vi "niUSRP EX Rx Continuous Async.vi"() -> ()   [LabVIEW 2020]
doc: "Continuously acquires a communication signal that starts immediately. The device is not synchronized to external Reference Clocks or timebases."
uses:
  <instrlib>/niUSRP/niUSRP Timestamp.ctl
  <extravilib>/ChannelInstances/High Speed Stream-a[.](cdb)/_Read For Replicate.vi
  <extravilib>/ChannelInstances/High Speed Stream-a[.](cdb)/Instantiate.vi
  <extravilib>/ChannelInstances/High Speed Stream-a[.](cdb)/)Channel.vi
  <extravilib>/ChannelInstances/High Speed Stream-a[.](cdb)/Abort Signal/Init Signal.vi
  <instrlib>/niUSRP/niUSRP Fetch Rx Data (CDB WDT).vi
  <vilib>/measure/maspectr.llb/FFT Power Spectrum for 1 Chan (CDB).vi
  <vilib>/measure/NI_MAPro.lvlib
  <extravilib>/ChannelInstances/High Speed Stream-a[.](cdb).lvlib
panel:
  out "size(s)":i32
  out "element":cdb[](array[numeric])
  out "error out":errorcluster
  in  "Enabled Channel":string="0"
  out "Actual Rx Timestamp":T1
  in  "Stop":bool
  in  "Device Name":refnum<k15>="192.168.10.2"
  in  "Active Antenna":string="RX1"
  out "Baseband Power Spectrum":cluster{"f0":dbl, "df":dbl, "magnitude":dbl[]}(graph)
  in  "Timeout":dbl=10.0 format="%#.3ps"
  in  "Number of Samples":i64=16384
  out "IQ Graph":waveform(dbl)[](graph)
  out "Coerced Gain":dbl format="%#_6f"
  out "Coerced Carrier Frequency":dbl=100000.0 format="%#_6p"
  out "Coerced IQ Rate [S/sec]":dbl=100000.0 format="%#_6p"
  in  "Gain":dbl=1.0 format="%#_6f"
  in  "Carrier Frequency":dbl=2000000000.0 format="%#_6p"
  in  "IQ Rate [S/sec]":dbl=1000000.0 format="%#_6p"
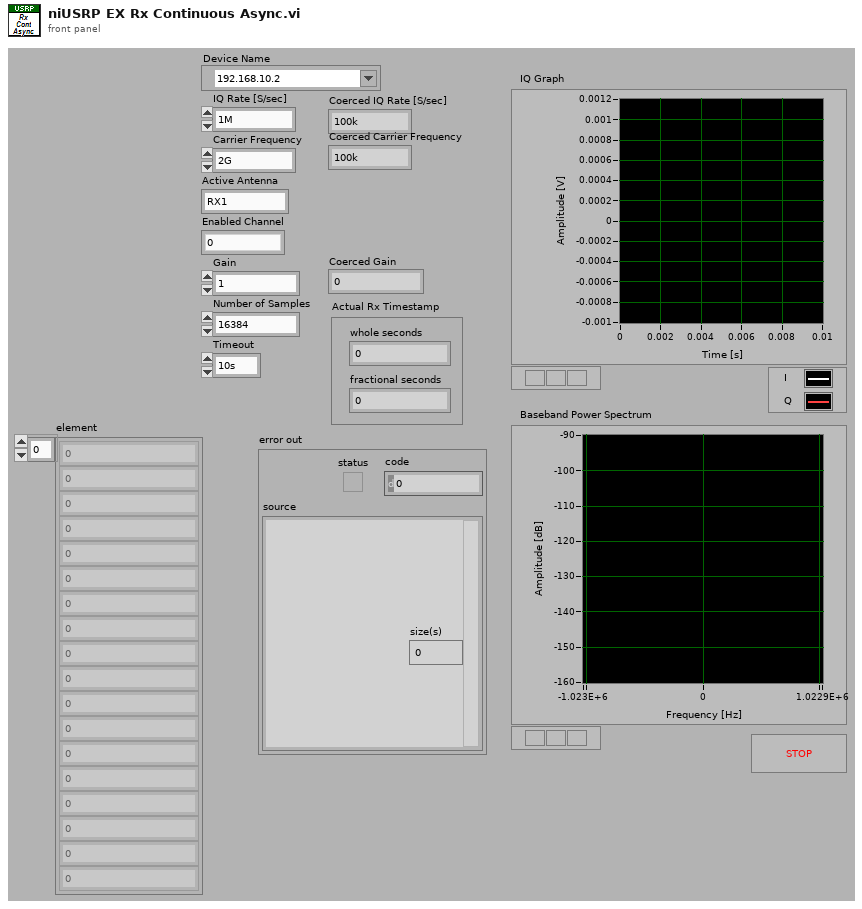
[diagram p1: front panel]
types:
  T1 = typedef "niUSRP Timestamp.ctl" = cluster{"whole seconds":u64, "fractional seconds":dbl}
  T2 = typedef "High Speed Stream-a[.](cdb).lvlib/)Channel.ctl" = refnum<queue>
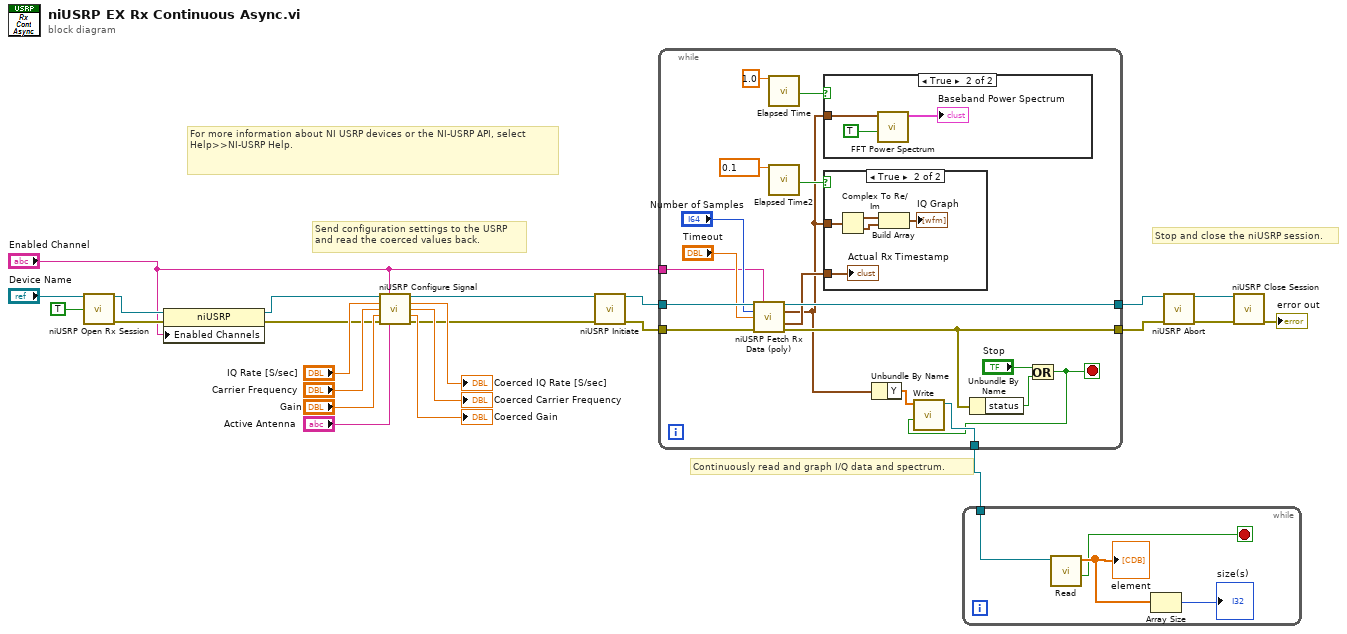
[diagram p0: block diagram]
diagram:
  # "For more information about NI USRP devices or the NI-USRP API, select Help>>NI-USRP Help."
  # "Stop and close the niUSRP session."
  # "Continuously read and graph I/Q data and spectrum."
  # "Send configuration settings to the USRP\nand read the coerced values back."
  n1 = call <instrlib>:"niUSRP Open Rx Session.vi"("device names"="Device Name", "reset"=TRUE) -> ("session handle out"=w8:refnum<k15>, "error out"=w6:errorcluster)  [unwired: 12 in]
  n2 = property class="niUSRP"(reference=w8, error in=w6, "Enabled Channels"="Enabled Channel") -> (reference out=w7:refnum<k15>, error out=w5:errorcluster)
  n3 = call <instrlib>:"niUSRP Configure Signal.vi"("session handle"=w7, "channel list"="Enabled Channel", "IQ rate"="IQ Rate [S/sec]", "carrier frequency"="Carrier Frequency", "gain"="Gain", "error in (no error)"=w5, "active antenna"="Active Antenna") -> ("session handle out"=w10:refnum<k15>, "coerced IQ rate"=→"Coerced IQ Rate [S/sec]":dbl, "coerced carrier frequency"=→"Coerced Carrier Frequency":dbl, "coerced gain"=→"Coerced Gain":dbl, "error out"=w9:errorcluster)  [unwired: 4 in]
  n4 = call <instrlib>:"niUSRP Initiate.vi"("session handle"=w10, "error in (no error)"=w9) -> ("session handle out"=w24:refnum<k15>, "error out"=w23:errorcluster)  [unwired: 12 in]
  n5 = while {
    tunnel: w24 -> [w42]
    tunnel: [w38] -> w22
    tunnel: "Enabled Channel" -> [w34]
    tunnel: w23 -> [w41]
    tunnel: [w37] -> w21
    tunnel: [w26] -> w1
    stop <- w25 stop-if-true
    n6 = call-poly <instrlib>:"niUSRP Fetch Rx Data (poly).vi"("session handle"=w42, "channel list"=w34, "number of samples"="Number of Samples", "timeout"="Timeout", "error in (no error)"=w41) -> ("session handle out"=w38:refnum<k15>, "data"=w28:waveform(cdb), "timestamp"=w31:T1, "error out"=w37:errorcluster)  [unwired: 7 in]
    n7 = call "Elapsed Time"("Time Target (s)"=1.0) -> ("Time has Elapsed"=w33:bool)  [unwired: 11 in, 7 out]
    n8 = call "Elapsed Time2"("Time Target (s)"=0.1) -> ("Time has Elapsed"=w32:bool)  [unwired: 11 in, 7 out]
    n9 = case shown="True" w33 {
      tunnel: w28 -> [_ w48]
      frame False {
      }
      frame True {
        n10 = call-poly <vilib>:"FFT Power Spectrum.vi"("dB On (F)"=TRUE, "time signal"=w48) -> ("power spectrum"=→"Baseband Power Spectrum":cluster{"f0":dbl, "df":dbl, "magnitude":dbl[]})  [unwired: 6 in, 3 out]
      }
    }
    n11 = case shown="True" w32 {
      tunnel: w28 -> [_ w44]
      tunnel: w31 -> [_ w43]
      frame False {
      }
      frame True {
        n12 = Complex To Re/Im(x + iy=w44) -> (x=w45:waveform(dbl), y=w46:waveform(dbl))
        n13 = Build Array(w45, w46) -> (→"IQ Graph":waveform(dbl)[])
        "Actual Rx Timestamp" <- w43
      }
    }
    n14 = Unbundle By Name(w28) -> ("Y"=w27:cdb[])
    n15 = Unbundle By Name(w37) -> ("status"=w35:bool)
    n16 = Or(x="Stop", y=w35) -> (x .or. y?=w25:bool)
    n17 = call <extravilib>:"Write.vi"("last element? (F)"=w25, "element"=w27) -> ("channel"=w26:T2)  [unwired: 7 in, 2 out]
  }
  n18 = while {
    tunnel: w1 -> [w54]
    stop <- w51 stop-if-true
    n19 = call <extravilib>:"Read.vi"("channel"=w54) -> ("done?"=w51:bool, "element"=w53:cdb[])  [unwired: 6 in, 3 out]
    "element" <- w53
    n20 = Array Size(array=w53) -> (size(s)=→"size(s)":i32)
  }
  n21 = call <instrlib>:"niUSRP Abort.vi"("session handle"=w22, "error in (no error)"=w21) -> ("session handle out"=w19:refnum<k15>, "error out"=w20:errorcluster)  [unwired: 12 in]
  n22 = call <instrlib>:"niUSRP Close Session.vi"("session handle"=w19, "error in (no error)"=w20) -> ("error out"=→"error out":errorcluster)  [unwired: 13 in]
